vi "myRIO_BRig_Host_formatData_convert__idx_to_colLetter.vi"(11 "input_idx":i32) -> (2 "output_colLetter":string)   [LabVIEW 2014]
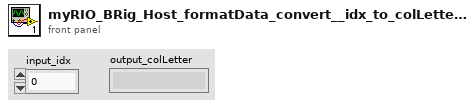
[diagram p1: front panel]
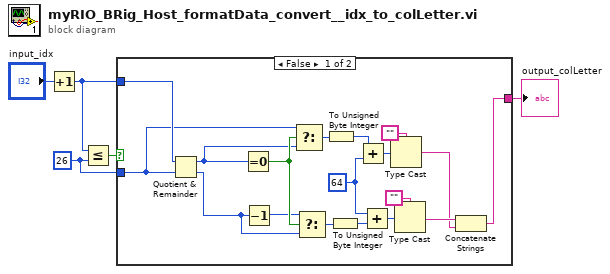
[diagram p0: block diagram]
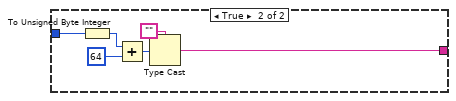
[diagram p2: hidden frame]
diagram:
  w2 = 26 ("y")
  n1 = Increment(x="input_idx") -> (x+1=w3:i32)
  n2 = Less Or Equal?(x=w3, y=w2) -> (x <= y?=w5:bool)
  n3 = case shown="False" w5 {
    tunnel: w3 -> [w23 w27]
    tunnel: w2 -> [w17 _]
    tunnel: [w6 w24] -> w1
    frame False {
      w9 = u8 64 ("y")
      n4 = Quotient & Remainder(x=w23, y=w17) -> (x-y*floor(x/y)=w21:i32, floor(x/y)=w19:i32)
      n5 = Equal To 0?(x=w21) -> (x = 0?=w22:bool)
      n6 = Decrement(x=w19) -> (x-1=w20:i32)
      n7 = Select(t=w17, s=w22, f=w21) -> (s? t:f=w11:i32)
      n8 = Select(t=w20, s=w22, f=w19) -> (s? t:f=w16:i32)
      n9 = To Unsigned Byte Integer(number=w11) -> (unsigned 8bit integer=w13:u8)
      n10 = To Unsigned Byte Integer(number=w16) -> (unsigned 8bit integer=w10:u8)
      n11 = Add(x=w13, y=w9) -> (x+y=w12:u8)
      n12 = Add(x=w9, y=w10) -> (x+y=w15:u8)
      n13 = Type Cast(type="", x=w12) -> (*(type *) &x=w7:string)
      n14 = Type Cast(type="", x=w15) -> (*(type *) &x=w8:string)
      n15 = Concatenate Strings(w8, w7) -> (w6:string)
    }
    frame True {
      n16 = To Unsigned Byte Integer(number=w27) -> (unsigned 8bit integer=w26:u8)
      n17 = Add(x=w26, y=u8 64) -> (x+y=w25:u8)
      n18 = Type Cast(type="", x=w25) -> (*(type *) &x=w24:string)
    }
  }
  "output_colLetter" <- w1
